vi "GetSetTriggerSource.vi"(7 "Set":bool, 8 "error in (no error)":errorcluster, 10 "Source":string, 11 "Data Value Reference in":refnum<data-value>) -> (0 "error out":errorcluster, 3 "Source":string)   [LabVIEW 2020, in "Camera.lvclass"]
uses:
  Camera.lvclass
  Camera.lvclass/Camera.ctl
  bin/gindustrialcam_32-1.dll
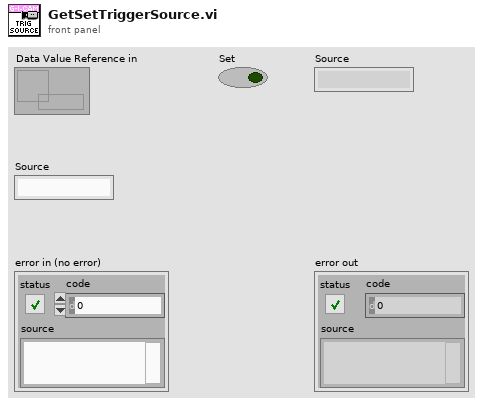
[diagram p1: front panel]
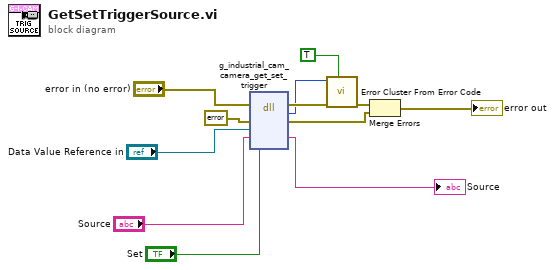
[diagram p0: block diagram]
diagram:
  n1 = dll-call lib="C:/serenial/lib/g-industrial-camera/LabVIEW/g_industrial_cam/bin/gindustrialcam_*-1.*" fn="g_industrial_cam_camera_get_set_trigger"(error in="error in (no error)", "err"=errorcluster {"status"=FALSE, "code"=0, "source"=""} ("error constant"), "edvr"="Data Value Reference in", "formats"="Source", "set"="Set") -> (error out=w11:errorcluster, "Mg_Error"=w10:i32, "err"=w8:errorcluster, "formats"=→"Source":string)  [unwired: 4 in, 1 out]
  n2 = call <vilib>:"Error Cluster From Error Code.vi"("show call chain? (False)"=TRUE, "error in (no error)"=w11, "error code (0)"=w10) -> ("error out"=w9:errorcluster)  [unwired: 6 in]
  n3 = Merge Errors(w9, w8) -> (→"error out":errorcluster)
